vi "Master network read write.vi"(8 "error in (no error)":errorcluster, 9 "Modbus Data Unit":T1={"function"=1, "Data"=[]} {"function" items=["Read Discrete Inputs"=2, "Read Coils"=1, "Write Single Coil"=5, "Write Multiple Coils"=15, "Read Input Register"=4, "Read Holding Registers"=3, "Write Single Register"=6, "Write Multiple Registers"=16, "Read/Write Multiple Registers"=23, "Mask Write Register"=22, "Read FIFO Queue"=24, "Read File Record"=20, "Write File Record"=21, "Read Exception Status"=7, "Diagnostic"=8, "Get Com Event Counter"=11, "Get Com Event Log"=12, "Report Slave ID"=17, "Read Device Identification"=43]; "Data" format="%.0x"}, 10 "Unit_ID":T3, 11 "TCP in":refnum<class "TCP.lvclass">) -> (0 "error out":errorcluster, 1 "Modbus data unit out":T1={"function"=1, "Data"=[]} {"function" items=["Read Discrete Inputs"=2, "Read Coils"=1, "Write Single Coil"=5, "Write Multiple Coils"=15, "Read Input Register"=4, "Read Holding Registers"=3, "Write Single Register"=6, "Write Multiple Registers"=16, "Read/Write Multiple Registers"=23, "Mask Write Register"=22, "Read FIFO Queue"=24, "Read File Record"=20, "Write File Record"=21, "Read Exception Status"=7, "Diagnostic"=8, "Get Com Event Counter"=11, "Get Com Event Log"=12, "Report Slave ID"=17, "Read Device Identification"=43]; "Data" format="%.0x"}, 3 "TCP out":refnum<class "TCP.lvclass">, 5 "PDU valid?":bool)   [LabVIEW 2021, in "NI_modbus_upd.lvlib"]
doc: "This VI allows a mutex for the master API without restricting any other functions. This mutex is currently unimplemented."
uses:
  NI_modbus_upd.lvlib
  Ctl/MB Modbus Data Unit.ctl
  Modbus Data Unit (PDU)/Function.ctl
  TCP/TCP.lvclass
  Ctl/Unit_ID.ctl
  TCP/TCP.lvclass/TCP.ctl
  Modbus Data Unit (PDU)/Unflatten to PDU1.vi
  TCP/Protocol Read.vi
  TCP/Protocol Write.vi
  <vilib>/Utility/error.llb/Clear Errors.vi
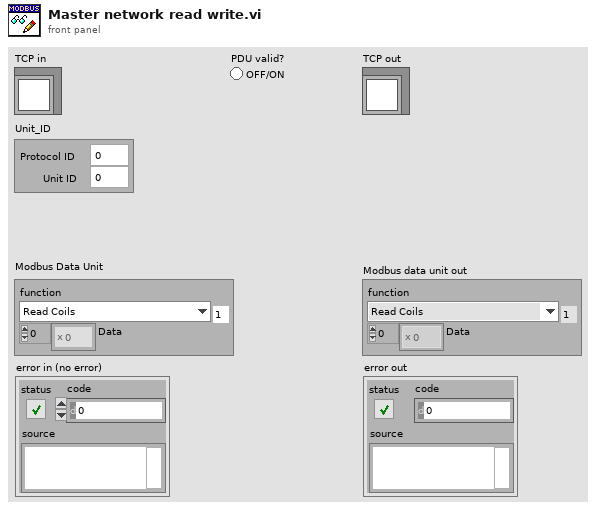
[diagram p1: front panel]
types:
  T1 = typedef "NI_modbus_upd.lvlib/MB Modbus Data Unit.ctl" = cluster{"function":T2, "Data":u8[]}
  T2 = typedef "NI_modbus_upd.lvlib/Function.ctl" = u8
  T3 = typedef "NI_modbus_upd.lvlib/Unit_ID.ctl" = cluster{"Protocol ID":u16, "Unit ID":u8}
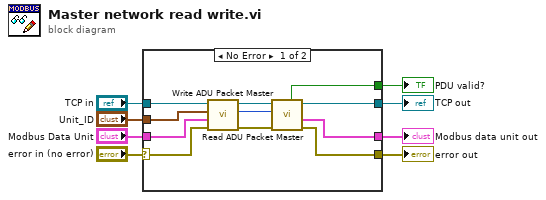
[diagram p0: block diagram]
diagram:
  n1 = case shown="No Error" "error in (no error)" {
    selector: "error in (no error)" -> [w16 w22]
    tunnel: "TCP in" -> [w19 w21]
    tunnel: [w18 w20] -> w8
    tunnel: [w9 w22] -> w7
    tunnel: [w17 _] -> w6
    tunnel: [w15 w21] -> w1
    tunnel: "Unit_ID" -> [w11 _]
    tunnel: "Modbus Data Unit" -> [w10 w20]
    frame No Error {
      n2 = call "Write ADU Packet Master.vi"("error in (no error) 2"=w16, "Modbus Data Unit"=w10, "Unit_ID"=w11, "TCP in"=w19) -> ("error out 2"=w14:errorcluster, "Transaction ID"=w12:u16, "TCP out"=w13:refnum<class "TCP.lvclass">)  [unwired: 5 in]
      n3 = call "Read ADU Packet Master.vi"("error in (no error)"=w14, "Transaction ID"=w12, "TCP in"=w13) -> ("error out"=w9:errorcluster, "Modbus Data Unit"=w18:T1, "TCP out"=w15:refnum<class "TCP.lvclass">, "PDU Valid?"=w17:bool)  [unwired: 5 in]
    }
    frame Error {
    }
  }
  "Modbus data unit out" <- w8
  "error out" <- w7
  "PDU valid?" <- w6
  "TCP out" <- w1
